vi "CheckFile.vi"(11 "Image count filepath":path) -> (3 "Byte Stream File out":refnum<file>)   [LabVIEW 2019]
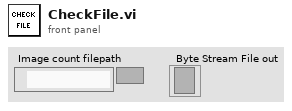
[diagram p1: front panel]
types:
  T1 = enum16{"open", "replace", "create", "open or create", "replace or create", "replace or create with confirmation"}
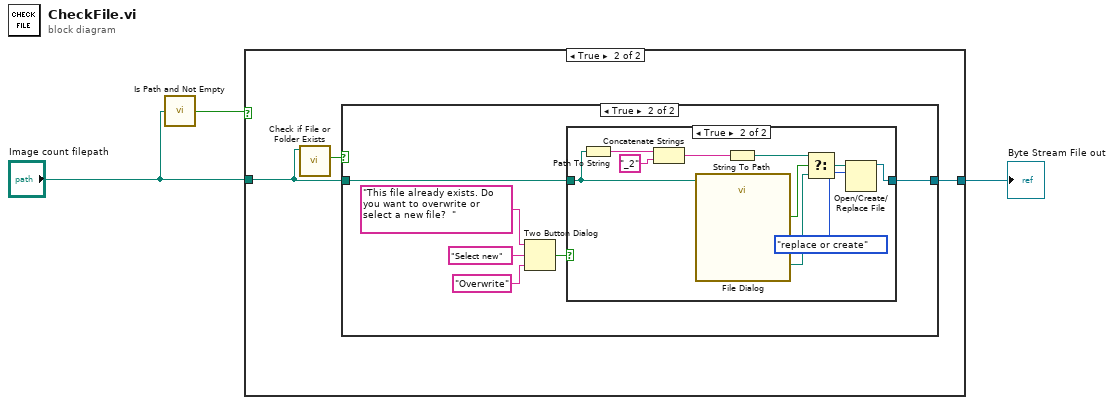
[diagram p0: block diagram]
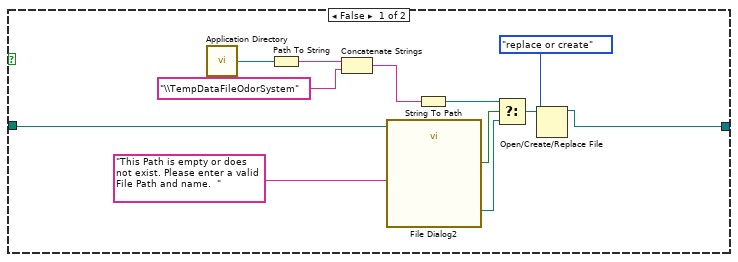
[diagram p2: hidden frame]
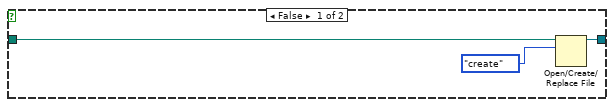
[diagram p3: hidden frame]
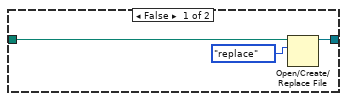
[diagram p4: hidden frame]
diagram:
  n1 = call <vilib>:"Is Path and Not Empty.vi"("path"="Image count filepath") -> ("Is Path and Not Empty?"=w2:bool)  [unwired: 4 in]
  n2 = case shown="True" w2 {
    tunnel: "Image count filepath" -> [w15 w17]
    tunnel: [w6 w16] -> w1
    frame False {
      n3 = call <vilib>:"Application Directory.vi"() -> ("Application Directory"=w5:path)
      n4 = Path To String(path=w5) -> (string=w8:string)
      n5 = Concatenate Strings(w8, "\\TempDataFileOdorSystem") -> (w10:string)
      n6 = call "File Dialog2"("start path"=w15, "prompt"="This Path is empty or does not exist. Please enter a valid File Path and name.  " ("message")) -> ("selected path"=w13:path, "cancelled"=w14:bool)  [unwired: 10 in, 2 out]
      n7 = String To Path(string=w10) -> (path=w9:path)
      n8 = Select(t=w9, s=w14, f=w13) -> (s? t:f=w12:path)
      n9 = Open/Create/Replace File(file path (use dialog)=w12, operation (0:open)=T1."replace or create") -> (refnum out=w6:refnum<file>)  [unwired: 4 in, 2 out]
    }
    frame True {
      n10 = call <vilib>:"Check if File or Folder Exists.vi"("path"=w17) -> ("file or folder exists?"=w18:bool)  [unwired: 8 in, 2 out]
      n11 = case shown="True" w18 {
        tunnel: w17 -> [w21 w22]
        tunnel: [w20 w27] -> w16
        frame False {
          n12 = Open/Create/Replace File(file path (use dialog)=w21, operation (0:open)=T1."create") -> (refnum out=w20:refnum<file>)  [unwired: 4 in, 2 out]
        }
        frame True {
          n13 = Two Button Dialog(message="This file already exists. Do you want to overwrite or select a new file?  ", 1:"Overwrite" ("F button name (\"Cancel\")"), 2:"Select new" ("T button name (\"OK\")")) -> (T button?=w23:bool)
          n14 = case shown="True" w23 {
            tunnel: [w30 w40] -> w27
            tunnel: w22 -> [w29 w32]
            frame False {
              n15 = Open/Create/Replace File(file path (use dialog)=w29, operation (0:open)=T1."replace") -> (refnum out=w30:refnum<file>)  [unwired: 4 in, 2 out]
            }
            frame True {
              n16 = Path To String(path=w32) -> (string=w33:string)
              n17 = Concatenate Strings(w33, "_2") -> (w35:string)
              n18 = call "File Dialog"("start path"=w32) -> ("selected path"=w38:path, "cancelled"=w39:bool)  [unwired: 11 in, 2 out]
              n19 = String To Path(string=w35) -> (path=w34:path)
              n20 = Select(t=w34, s=w39, f=w38) -> (s? t:f=w37:path)
              n21 = Open/Create/Replace File(file path (use dialog)=w37, operation (0:open)=T1."replace or create") -> (refnum out=w40:refnum<file>)  [unwired: 4 in, 2 out]
            }
          }
        }
      }
    }
  }
  "Byte Stream File out" <- w1
